vi "ConfigureOutput.vi"(8 "error in (no error)":errorcluster, 10 "Output((F)":bool, 11 "YP03-60_Z in":refnum<class "YP03-60_Z.lvclass">) -> (0 "error out":errorcluster, 3 "YP03-60_Z out":refnum<class "YP03-60_Z.lvclass">)   [LabVIEW 2020, in "PowerControl.lvlib" / "YP03-60_Z.lvclass"]
uses:
  YP03-60_Z.lvclass
  YP03-60_Z.lvclass/YP03-60_Z.ctl
  <vilib>/Instr/_visa.llb/VISA Configure Serial Port (Instr).vi
  VirtualPower/VirtualPower.lvclass
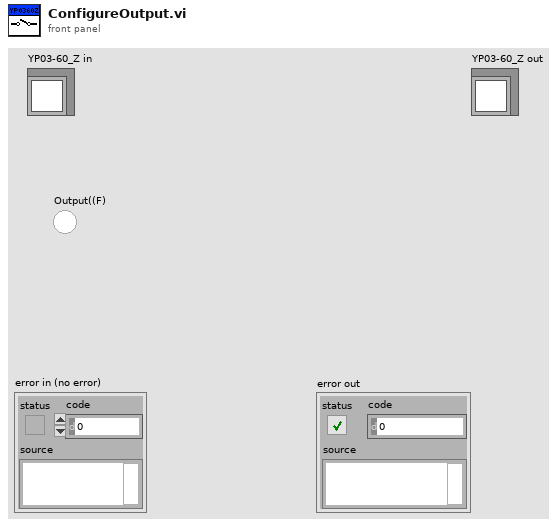
[diagram p1: front panel]
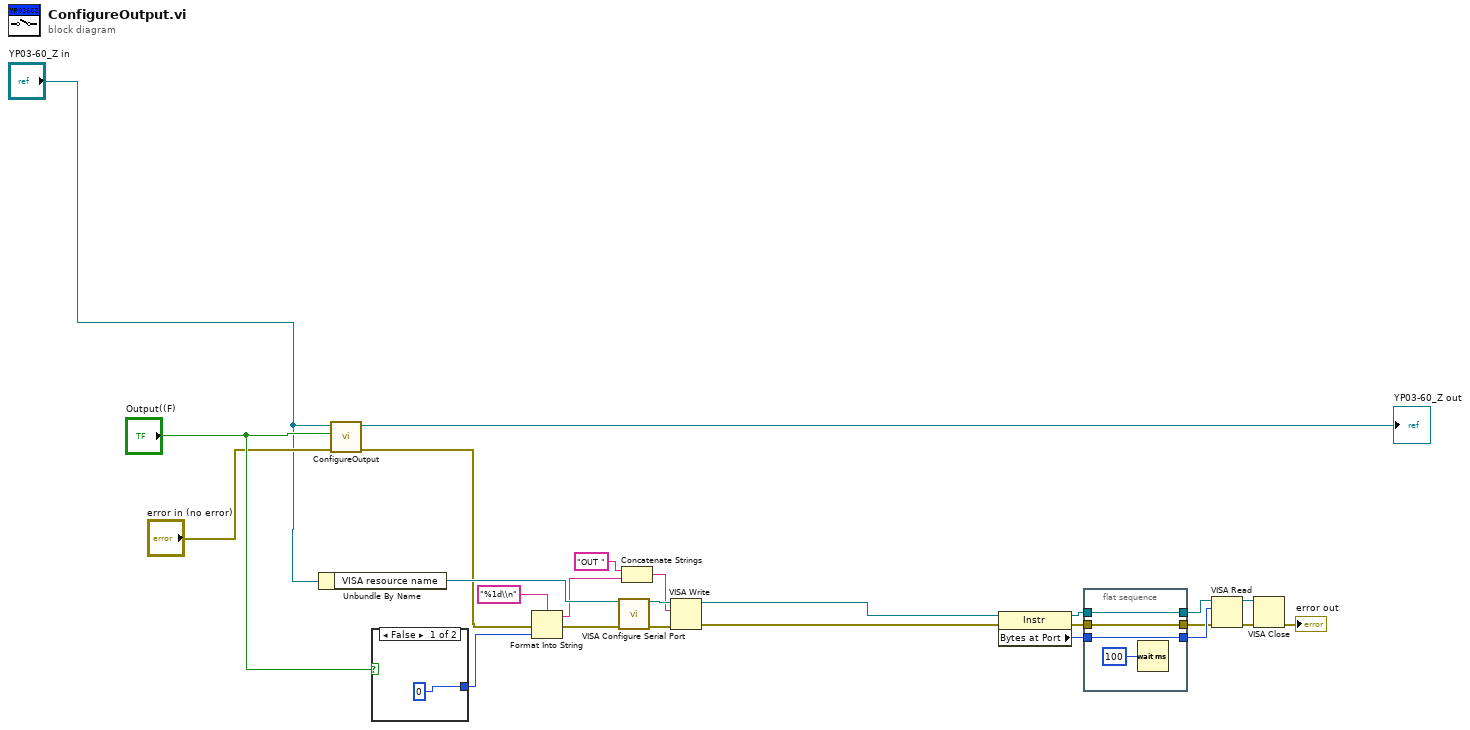
[diagram p0: block diagram]
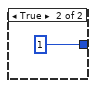
[diagram p2: hidden frame]
diagram:
  n1 = Unbundle By Name("YP03-60_Z in") -> ("VISA resource name"=w21:refnum<visa-resource-name>)
  n2 = call-parent "ConfigureOutput.vi"("error in (no error)"="error in (no error)", "Output((F)"="Output((F)", "VirtualPower in"="YP03-60_Z in") -> ("error out"=w16:errorcluster, "VirtualPower out"=→"YP03-60_Z out":refnum<class "YP03-60_Z.lvclass">)  [unwired: 7 in]
  n3 = case shown="False" "Output((F)" {
    tunnel: [0 1] -> w25
    frame False {
    }
    frame True {
    }
  }
  n4 = Format Into String(format string="%1d\\n", error in=w16, w25) -> (resulting string=w13:string, error out=w18:errorcluster)  [unwired: 1 in]
  n5 = call-poly "VISA Configure Serial Port"("VISA resource name"=w21, "error in (no error)"=w18) -> ("VISA resource name out"=w20:refnum<visa-resource-name>, "error out"=w19:errorcluster)  [unwired: 12 in]
  n6 = Concatenate Strings("OUT " ("string"), w13) -> (w10:string)
  n7 = VISA Write(VISA resource name=w20, write buffer=w10, error in (no error)=w19) -> (VISA resource name out=w12:refnum<visa-resource-name>, error out=w11:errorcluster)  [unwired: 1 out]
  n8 = property class="Instr"(reference=w12, error in=w11) -> (reference out=w7:refnum<visa-resource-name>, error out=w5:errorcluster, "Bytes at Port"=w9:u32)
  n9 = flat-sequence {
    tunnel: w7 -> [w31]
    tunnel: [w31] -> w6
    tunnel: [w30] -> w4
    tunnel: w5 -> [w30]
    tunnel: [w29] -> w8
    tunnel: w9 -> [w29]
    frame #0 {
      n10 = Wait (ms)(milliseconds to wait=u32 100) -> ()  [unwired: 1 out]
    }
  }
  n11 = VISA Read(VISA resource name=w6, byte count=w8, error in (no error)=w4) -> (VISA resource name out=w24:refnum<visa-resource-name>, error out=w22:errorcluster)  [unwired: 2 out]
  n12 = VISA Close(VISA resource name=w24, error in (no error)=w22) -> (error out=→"error out":errorcluster)
